vi "Read File Path.vi"(8 "error in (no error)":errorcluster, 11 "Read in":refnum<class "Read.lvclass">) -> (0 "error out":errorcluster, 2 "File Ref":refnum<file>, 3 "Read out":refnum<class "Read.lvclass">)   [LabVIEW 2014, in "Read.lvclass"]
uses:
  Read.lvclass
  Read.lvclass/Read.ctl
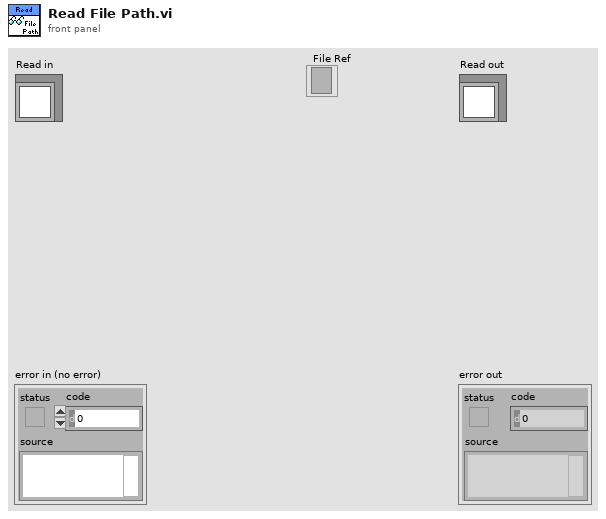
[diagram p1: front panel]
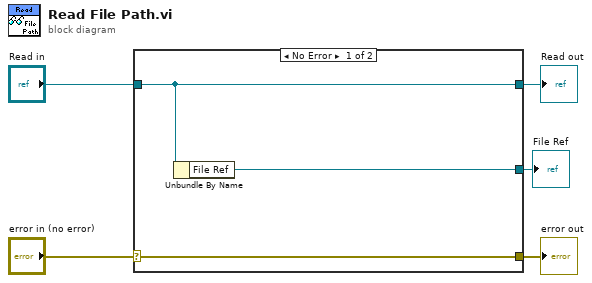
[diagram p0: block diagram]
diagram:
  n1 = case shown="No Error" "error in (no error)" {
    selector: "error in (no error)" -> [w8 w9]
    tunnel: [w8 w9] -> w4
    tunnel: [w7 w10] -> w2
    tunnel: "Read in" -> [w7 w10]
    tunnel: [w6 _] -> w1
    frame No Error {
      n2 = Unbundle By Name(w7) -> ("File Ref"=w6:refnum<file>)
    }
    frame Error {
    }
  }
  "error out" <- w4
  "Read out" <- w2
  "File Ref" <- w1
